vi "Write PhysicalChannels.vi"(8 "error in (no error)":errorcluster, 10 "PhysicalChannels":T1=["", "", "", "", "", "", "", "", ""], 11 "NiPxi6123 in":refnum<class "NiPxi6123.lvclass">) -> (0 "error out":errorcluster, 3 "NiPxi6123 out":refnum<class "NiPxi6123.lvclass">)   [LabVIEW 2014, in "SamplerPlugins.lvlib" / "NiPxi6123.lvclass"]
uses:
  NiPxi6123.lvclass
  TypeDefs/sPhysicalChannels.ctl
  NiPxi6123.lvclass/NiPxi6123.ctl
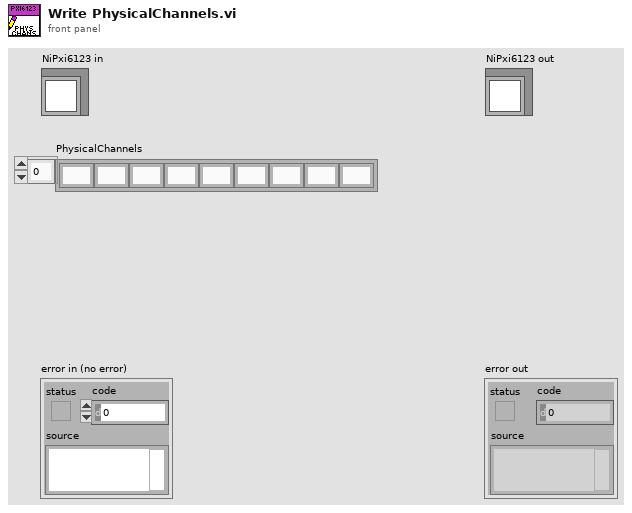
[diagram p1: front panel]
types:
  T1 = typedef "SamplerPlugins.lvlib/NiPxi6123.lvclass/sPhysicalChannels.ctl" = string[]
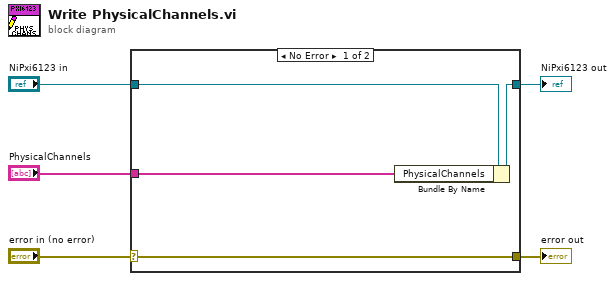
[diagram p0: block diagram]
diagram:
  n1 = case shown="No Error" "error in (no error)" {
    selector: "error in (no error)" -> [w9 w10]
    tunnel: [w9 w10] -> w4
    tunnel: [w7 w11] -> w2
    tunnel: "NiPxi6123 in" -> [w8 w11]
    tunnel: "PhysicalChannels" -> [w6 _]
    frame No Error {
      n2 = Bundle By Name(cluster=w8, "PhysicalChannels"=w6) -> (w7:refnum<class "NiPxi6123.lvclass">)
    }
    frame Error {
    }
  }
  "error out" <- w4
  "NiPxi6123 out" <- w2
